vi "Script_Extract_Wfms.vi"(7 "Script Text":string, 8 "error in (no error)":errorcluster, 10 "Script File":string="Pirenea2Excits1Acq4s.txt", 11 "Script Path":path=path "D:/PIRENEA/TECHNICAL/TIMING_SCRIPTS") -> (0 "error out":errorcluster, 2 "Script Text Cleaned":string, 3 "Table of Wfms":string[](array[string]))   [LabVIEW 2017]
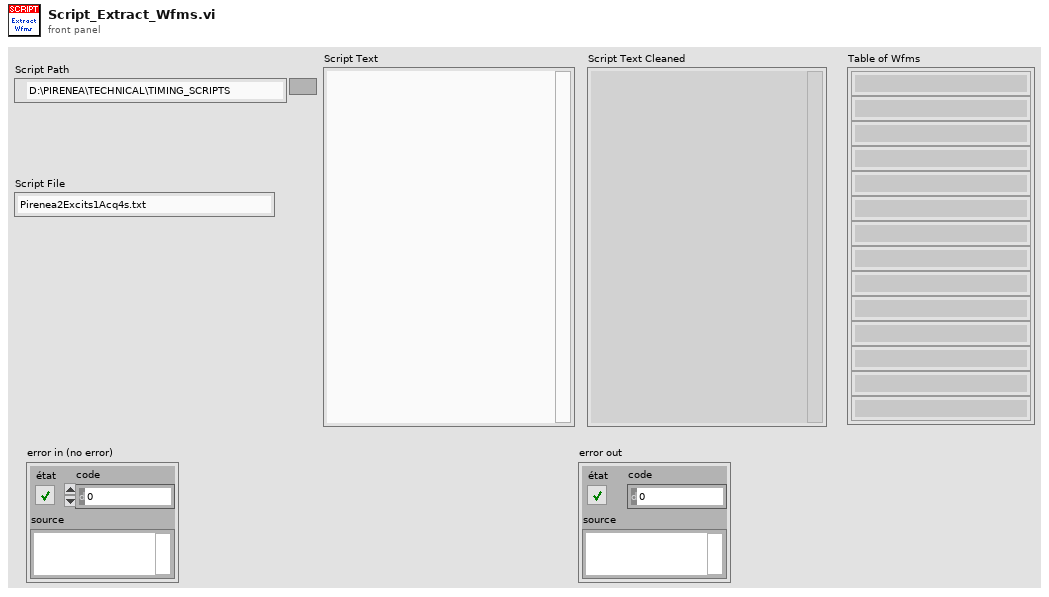
[diagram p1: front panel]
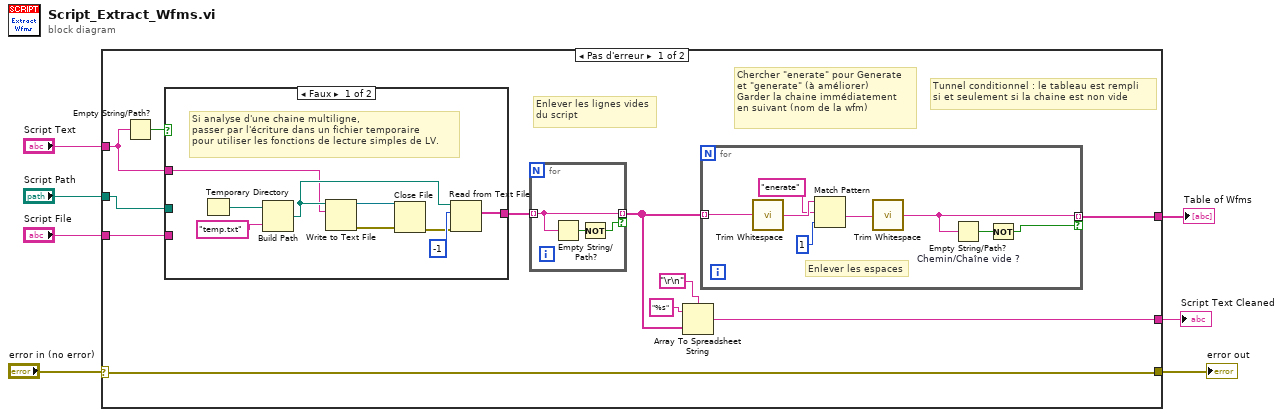
[diagram p0: block diagram]
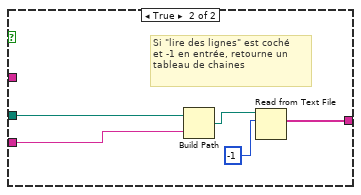
[diagram p2: hidden frame]
diagram:
  n1 = case shown="Pas d'erreur" "error in (no error)" {
    selector: "error in (no error)" -> [w8 w44]
    tunnel: [w17 _] -> w7
    tunnel: "Script Text" -> [w13 _]
    tunnel: [w11 _] -> w5
    tunnel: "Script Path" -> [w9 _]
    tunnel: "Script File" -> [w10 _]
    tunnel: [w8 w44] -> w2
    frame No Error {
      # "Enlever les lignes vides\ndu script"
      # "Tunnel conditionnel : le tableau est rempli\nsi et seulement si la chaine est non vide"
      # "Chercher \"enerate\" pour Generate\net \"generate\" (à améliorer)\nGarder la chaine immédiatement\nen suivant (nom de la wfm)"
      n2 = Empty String/Path?(string/path=w13) -> (empty?=w12:bool)
      n3 = case shown="Faux" w12 {
        tunnel: w10 -> [_ w35]
        tunnel: w9 -> [_ w34]
        tunnel: [w22 w31] -> w14
        tunnel: w13 -> [w23 _]
        frame False {
          # "Si analyse d'une chaine multiligne,\npasser par l'écriture dans un fichier temporaire\npour utiliser les fonctions de lecture simples de LV."
          n4 = Temporary Directory() -> (w29:path)
          n5 = Build Path(base path=w29, name or relative path="temp.txt" ("nom ou chemin relatif")) -> (appended path=w26:path)
          n6 = Write to Text File(file (use dialog)=w26, text=w23) -> (refnum out=w27:refnum<file>, error out=w28:errorcluster)  [unwired: 2 in, 1 out]
          n7 = Close File(refnum=w27, error in=w28) -> (error out=w24:errorcluster)  [unwired: 1 out]
          n8 = Read from Text File(file (use dialog)=w26, count=-1 ("nombre"), error in=w24) -> (text=w22:string[])  [unwired: 1 in, 3 out]
        }
        frame True {
          # "Si \"lire des lignes\" est coché\net -1 en entrée, retourne un tableau de chaines"
          n9 = Build Path(base path=w34, name or relative path=w35) -> (appended path=w33:path)
          n10 = Read from Text File(file (use dialog)=w33, count=-1 ("nombre")) -> (text=w31:string[])  [unwired: 2 in, 3 out]
        }
      }
      n11 = for {
        tunnel: w14 -> [w20] mode=indexing
        tunnel: [w20] -> w15 mode=indexing if=w19
        n12 = Empty String/Path?(string/path=w20) -> (empty?=w21:bool)
        n13 = Not(x=w21) -> (.not. x?=w19:bool)
      }
      n14 = Array To Spreadsheet String(delimiter (Tab)="\r\n", array=w15, 3:"%s" ("chaîne de format")) -> (spreadsheet string=w17:string)
      n15 = for {
        tunnel: w15 -> [w43] mode=indexing
        tunnel: [w36] -> w11 mode=indexing if=w37
        # "Enlever les espaces"
        n16 = call <vilib>:"Trim Whitespace.vi"("string"=w43) -> ("trimmed string"=w42:string)  [unwired: 1 in]
        n17 = Match Pattern(string=w42, regular expression="enerate" ("expression régulière"), offset (0)=1) -> (after substring=w39:string)  [unwired: 3 out]
        n18 = call <vilib>:"Trim Whitespace.vi"("string"=w39) -> ("trimmed string"=w36:string)  [unwired: 1 in]
        n19 = Empty String/Path? "Chemin/Chaîne vide ?"(string/path=w36) -> (empty?=w38:bool)
        n20 = Not(x=w38) -> (.not. x?=w37:bool)
      }
    }
    frame Error {
    }
  }
  "Script Text Cleaned" <- w7
  "Table of Wfms" <- w5
  "error out" <- w2
